vi "RFP_Concatenate.vi"(4 "Output Index":i32, 5 "Channel Values In":string[][](array[string]), 6 "Channel Names":string[](array[string]), 7 "Maths Equation":string) -> (0 "Error String":string, 1 "Channel Values Out":string[][](array[string]))   [LabVIEW 2021]
uses:
  Data_plotting_vis/Results_plotter_Global.vi
  <vilib>/Utility/error.llb/whitespace.ctl
panel:
  out "Generic Equation":string
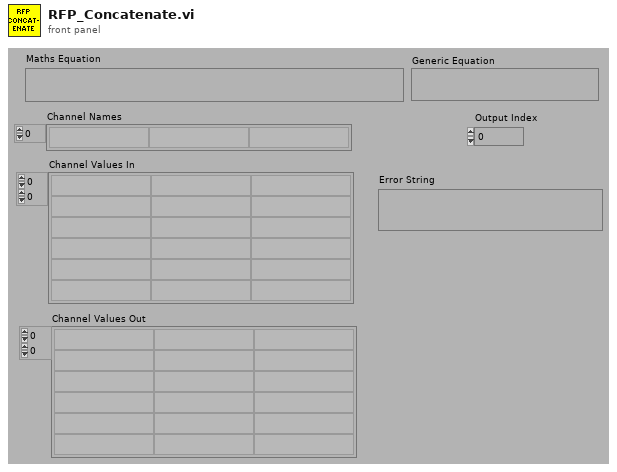
[diagram p1: front panel]
types:
  T1 = typedef "whitespace.ctl" = u16
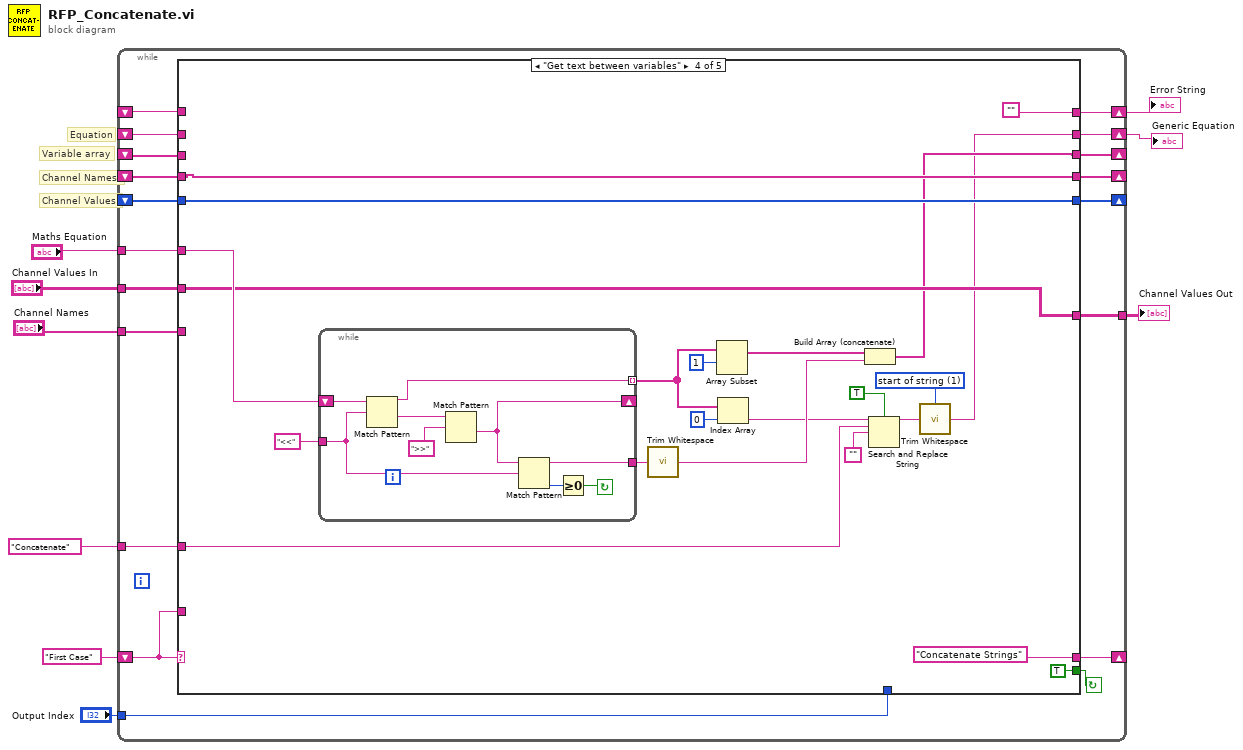
[diagram p0: block diagram]
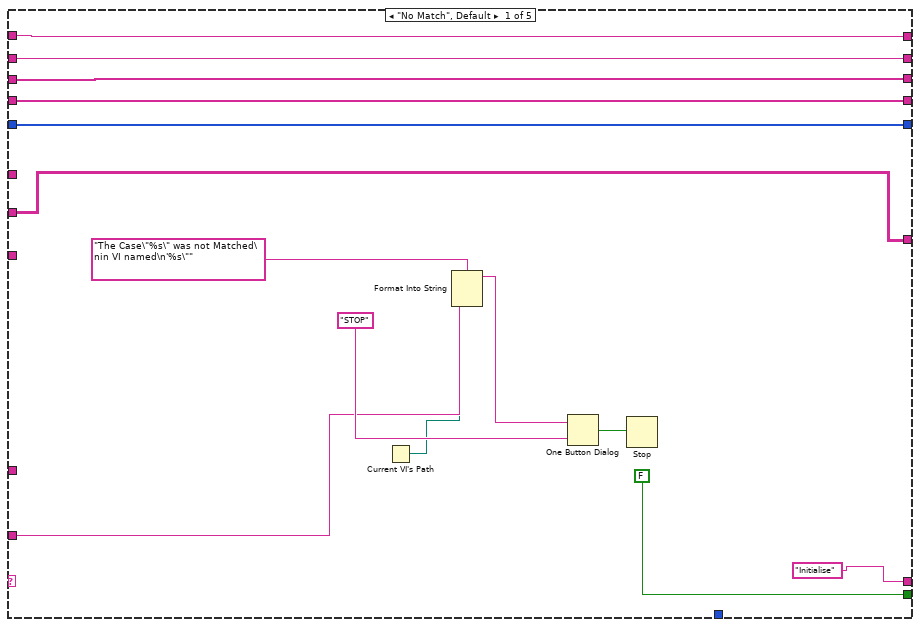
[diagram p2: hidden frame]
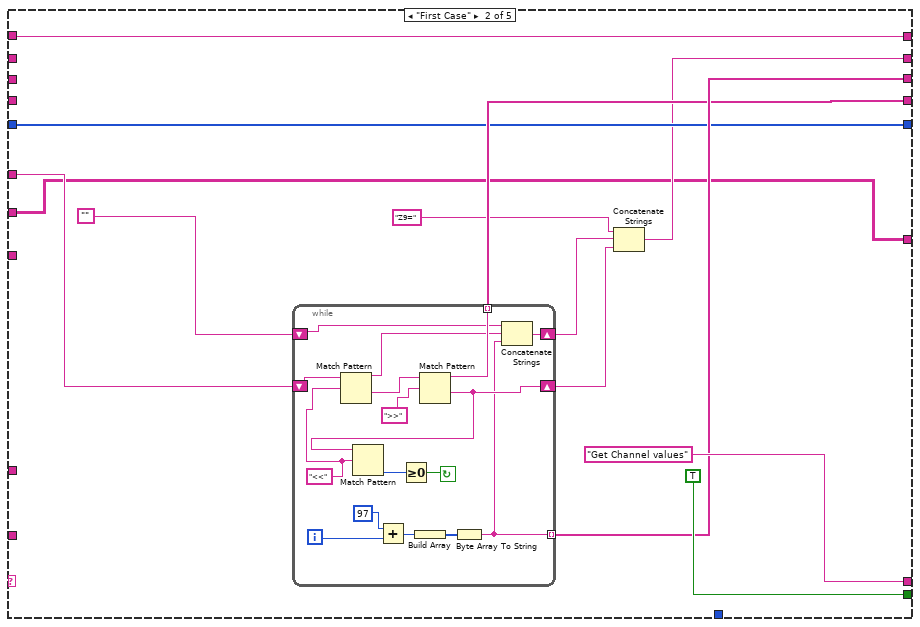
[diagram p3: hidden frame]
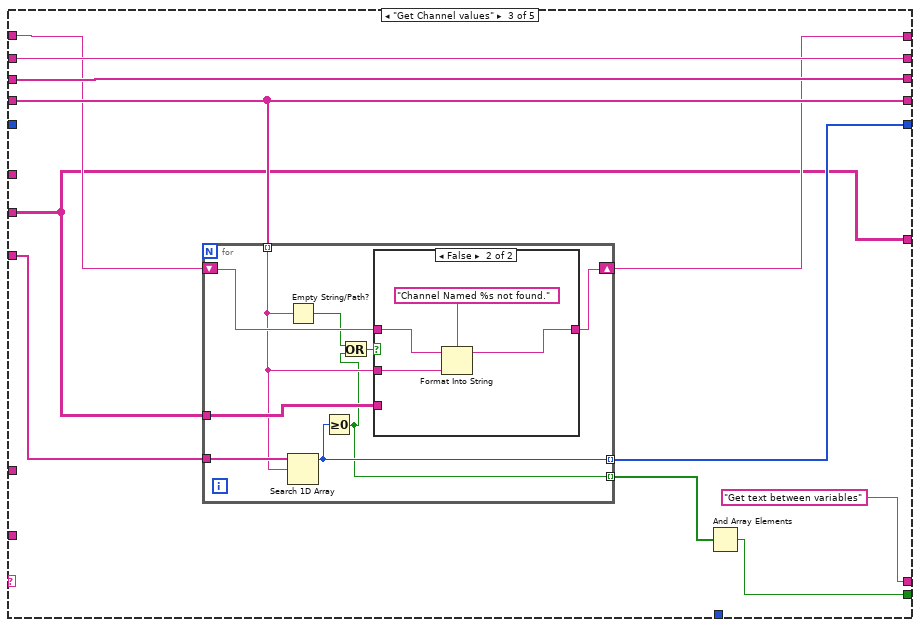
[diagram p4: hidden frame]
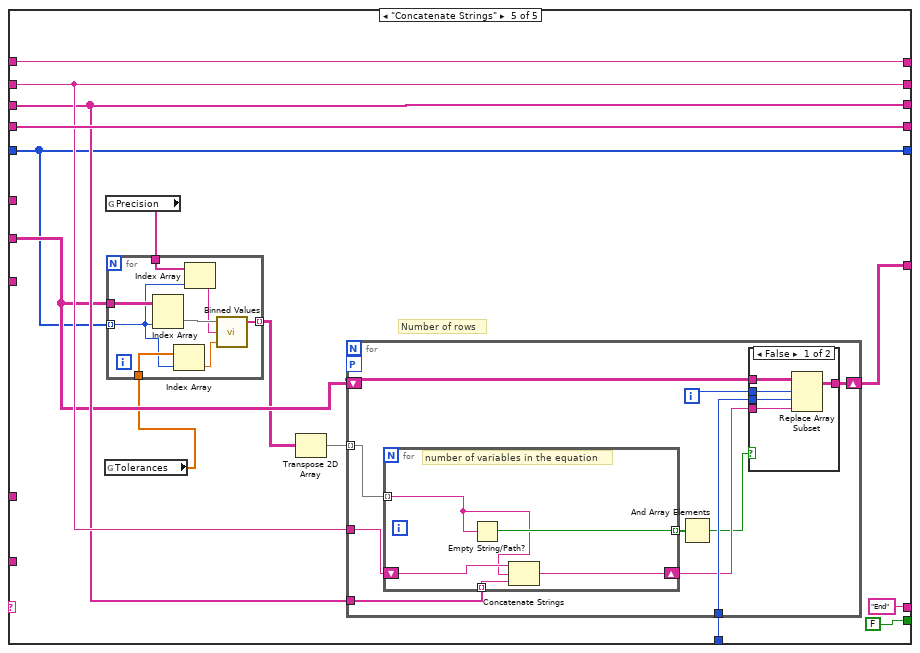
[diagram p6: hidden frame]
diagram:
  # "Channel Names"
  # "Variable array"
  # "Channel Values"
  # "Equation"
  n1 = while {
    tunnel: [w11] -> w3
    tunnel: "Output Index" -> [w12]
    tunnel: "Channel Values In" -> [w13]
    tunnel: "Channel Names" -> [w14]
    tunnel: "Maths Equation" -> [w15]
    shift-left: _ -> [w17]
    shift-right: [w16] -> _
    shift-left: _ -> [w19]
    shift-right: [w18] -> _
    shift-left: _ -> [w21]
    shift-right: [w20] -> _
    shift-left: _ -> [w23]
    shift-right: [w22] -> w5
    shift-left: _ -> [w25]
    shift-right: [w24] -> w6
    shift-left: "First Case" -> [w26]
    shift-right: [w27] -> _
    tunnel: "Concatenate" ("regular expression") -> [w10]
    stop <- w28 continue-if-true
    n2 = case shown="\"Get text between variables\"" w26 {
      tunnel: [FALSE TRUE w72 TRUE FALSE] -> w28
      tunnel: ["Initialise" "Get Channel values" "Get text between variables" "Concatenate Strings" "End"] -> w27
      tunnel: w26 -> [w37 _ _ _ _]
      tunnel: w25 -> [w34 w43 w76 _ w137]
      tunnel: [w34 w43 w77 "" w137] -> w24
      tunnel: w23 -> [w33 _ w82 _ w134]
      tunnel: [w33 w45 w82 w98 w134] -> w22
      tunnel: w21 -> [w32 _ w81 _ w133]
      tunnel: [w32 w52 w81 w107 w133] -> w20
      tunnel: w19 -> [w31 _ w79 w112 w138]
      tunnel: [w31 w48 w79 w112 w138] -> w18
      tunnel: w17 -> [w30 w47 _ w114 w131]
      tunnel: [w30 w47 w78 w114 w131] -> w16
      tunnel: w15 -> [_ w53 _ w116 _]
      tunnel: w14 -> [_ _ w80 _ _]
      tunnel: w13 -> [w29 w44 w75 w113 w132]
      tunnel: w12 -> [_ _ _ _ w136]
      tunnel: [w29 w44 w75 w113 w135] -> w11
      tunnel: w10 -> [_ _ _ w105 _]
      frame "No Match", Default {
        n3 = Current VI's Path() -> (path=w36:path)
        n4 = Format Into String(format string="The Case\"%s\" was not Matched\nin VI named\n'%s\"" ("Format String"), w37, w36) -> (resulting string=w40:string)  [unwired: 2 in, 1 out]
        n5 = One Button Dialog(message=w40, button name ("OK")="STOP") -> (true=w38:bool)
        n6 = Stop(stop? (T)=w38) -> ()
      }
      frame "First Case" {
        n7 = while {
          shift-left: "" -> [w58]
          shift-right: [w59] -> w50
          tunnel: [w60] -> w52 mode=indexing
          tunnel: [w66] -> w48 mode=indexing
          shift-left: w53 -> [w71]
          shift-right: [w69] -> w49
          i -> [w62]
          stop <- w67 continue-if-true
          w57 = "<<" ("regular expression")
          n8 = Match Pattern(string=w71, regular expression=w57) -> (before substring=w61:string, after substring=w70:string)  [unwired: 3 out]
          n9 = Add(x=97, y=w62) -> (x+y=w64:i32)
          n10 = Build Array(w64) -> (w65:i32[])
          n11 = Match Pattern(string=w70, regular expression=">>") -> (before substring=w66:string, after substring=w69:string)  [unwired: 3 out]
          n12 = Match Pattern(string=w69, regular expression=w57) -> (offset past match=w68:i32)  [unwired: 4 out]
          n13 = Greater Or Equal To 0?(x=w68) -> (x >= 0?=w67:bool)
          n14 = Byte Array To String(unsigned byte array=w65) -> (string=w60:string)
          n15 = Concatenate Strings(w58, w61, w60) -> (w59:string)
        }
        n16 = Concatenate Strings("Z9=" ("Substring"), w50, w49) -> (w45:string)
      }
      frame "Get Channel values" {
        n17 = for {
          tunnel: w80 -> [w91]
          tunnel: w79 -> [w86] mode=indexing
          tunnel: w75 -> [w90]
          tunnel: [w87] -> w78 mode=indexing
          shift-right: [w88] -> w77
          shift-left: w76 -> [w89]
          tunnel: [w84] -> w74 mode=indexing
          n18 = Empty String/Path?(string/path=w86) -> (empty?=w83:bool)
          n19 = Search 1D Array(1D array=w91, element=w86) -> (index of element=w87:i32)  [unwired: 1 out]
          n20 = Greater Or Equal To 0?(x=w87) -> (x >= 0?=w84:bool)
          n21 = Or(x=w83, y=w84) -> (x .or. y?=w85:bool)
          n22 = case shown="False" w85 {
            tunnel: w90 -> [_ _]
            tunnel: w86 -> [_ w96]
            tunnel: w89 -> [w92 w94]
            tunnel: [w92 w93] -> w88
            frame True {
            }
            frame False {
              n23 = Format Into String(format string="Channel Named %s not found." ("Format String"), initial string=w94, w96) -> (resulting string=w93:string)  [unwired: 1 in, 1 out]
            }
          }
        }
        n24 = And Array Elements(Boolean array=w74) -> (logical AND=w72:bool)
      }
      frame "Get text between variables" {
        w97 = T1 1 items=["both", "start of string", "end of string"] ("location (both)")
        n25 = while {
          shift-left: w116 -> [w126]
          shift-right: [w121] -> _
          tunnel: [w122] -> w110 mode=indexing
          tunnel: [w121] -> w104
          tunnel: "<<" ("regular expression") -> [w119]
          stop <- w123 continue-if-true
          n26 = Match Pattern(string=w126, regular expression=w119) -> (before substring=w122:string, after substring=w125:string)  [unwired: 3 out]
          n27 = Match Pattern(string=w125, regular expression=">>") -> (after substring=w121:string)  [unwired: 4 out]
          n28 = Match Pattern(string=w121, regular expression=w119) -> (offset past match=w124:i32)  [unwired: 4 out]
          n29 = Greater Or Equal To 0?(x=w124) -> (x >= 0?=w123:bool)
        }
        n30 = call <vilib>:"Trim Whitespace.vi"("string"=w104) -> ("trimmed string"=w106:string)  [unwired: 1 in]
        n31 = Array Subset(array=w110, index=1) -> (w109:string[])  [unwired: 1 in]
        n32 = Index Array(array=w110, index=0) -> (element=w102:string)
        n33 = Build Array (concatenate)(w109, w106) -> (w107:string[])
        n34 = Search and Replace String(case sensitive?=TRUE ("ignore case? (F)"), input string=w102, search string=w105, replace string="") -> (result string=w100:string)  [unwired: 4 in, 3 out]
        n35 = call <vilib>:"Trim Whitespace.vi"("string"=w100, "location (both)"=w97) -> ("trimmed string"=w98:string)
      }
      frame "Concatenate Strings" {
        # "Number of rows"
        n36 = global read "Results_plotter_Global.vi" "Tolerances"() -> (w127:dbl[])
        n37 = global read "Results_plotter_Global.vi" "Precision"() -> (w130:string[])
        n38 = for {
          tunnel: w132 -> [w148]
          tunnel: w131 -> [w143] mode=indexing
          tunnel: w130 -> [w146]
          tunnel: w127 -> [w144]
          tunnel: [w141] -> w129 mode=indexing
          n39 = Index Array(array=w148, index (col)=w143) -> (element=w147:string[])  [unwired: 1 in]
          n40 = Index Array(array=w144, index=w143) -> (element=w142:dbl)
          n41 = Index Array(array=w146, index=w143) -> (element=w145:string)
          n42 = call "Binned Values.vi"("Tolerance"=w142, "Precision (3)"=w145, "String Array In"=w147) -> ("String Array Out"=w141:string[])  [unwired: 2 in]
        }
        n43 = Transpose 2D Array(2D array=w129) -> (transposed array=w128:string[][])
        n44 = for {
          shift-right: [w157] -> w135
          shift-left: w132 -> [w158]
          tunnel: w136 -> [w155]
          tunnel: w134 -> [w154]
          tunnel: w133 -> [w153]
          tunnel: w128 -> [w149] mode=indexing
          workers-P: _ -> [_]
          i -> [w156]
          n45 = for {
            tunnel: w149 -> [w165] mode=indexing
            shift-right: [w167] -> w152
            shift-left: w154 -> [w169]
            tunnel: w153 -> [w168] mode=indexing
            tunnel: [w166] -> w151 mode=indexing
            # "number of variables in the equation"
            n46 = Empty String/Path?(string/path=w165) -> (empty?=w166:bool)
            n47 = Concatenate Strings(w169, w165, w168) -> (w167:string)
          }
          n48 = And Array Elements(Boolean array=w151) -> (logical AND=w150:bool)
          n49 = case shown="False" w150 {
            tunnel: w158 -> [w163 w164]
            tunnel: [w162 w164] -> w157
            tunnel: w156 -> [w161 _]
            tunnel: w155 -> [w160 _]
            tunnel: w152 -> [w159 _]
            frame False {
              n50 = Replace Array Subset(array=w163, new element=w159, index (row)=w161, index (col)=w160) -> (w162:string[][])
            }
            frame True {
            }
          }
        }
      }
    }
  }
  "Error String" <- w6
  "Generic Equation" <- w5
  "Channel Values Out" <- w3
